vi "Stepper Mover.vi"() -> ()   [LabVIEW 2018]
doc: "Use this template to build a producer/consumer design pattern with events to produce queue items. Use this design pattern instead of the User Interface Event Handler pattern for user interfaces when you want to execute code asynchronously in response to an event without slowing the user interface responsiveness."
uses:
  publisher action.ctl
panel:
  in  "Instrument Address":refnum<visa-resource-name>="ASRL2::INSTR"
  in  "Tab Control":enum32{"main", "ignore"}(tab)
  in  "move-to pos!":dbl(slide)=743.9484386624194 scale=0.0..10000.0 scale format="%^#6_6g"
  out "current pos...":dbl(slide) scale=0.0..10000.0
  in  "set velocity!":i32=1001
  in  "Stop!":bool
  out "Moving..":bool
  in  "Init!":bool
  in  "Set to zero!":bool
  out "error out":errorcluster={"status"=TRUE, "code"=5202, "source"="Stepper Command Match"}
  out "Current Bottom Position":dbl format="%.4f"
  in  "Move to Bottom Position (deg or in)":dbl=10.41515984909622 format="%.4f"
  in  "Rotator":T1(ring)=enum."System B 50 mm Magnet"
  out "Timeout error":bool
  in  "Exit!":bool
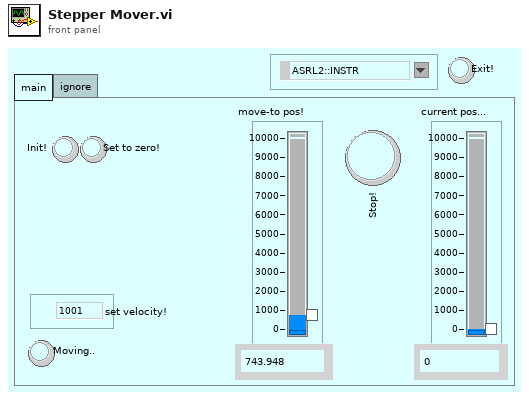
[diagram p1: front panel]
types:
  T1 = enum16{"Dilution Fridge SCM 1", "System A SCM 2", "System B 50 mm Magnet", "He-3 32 mm Magnet", "Portable Dil Fridge Rotator", "Linear Position", "System E Probe 1"}
  T2 = typedef "publisher action.ctl" = enum16{"set", "get"}
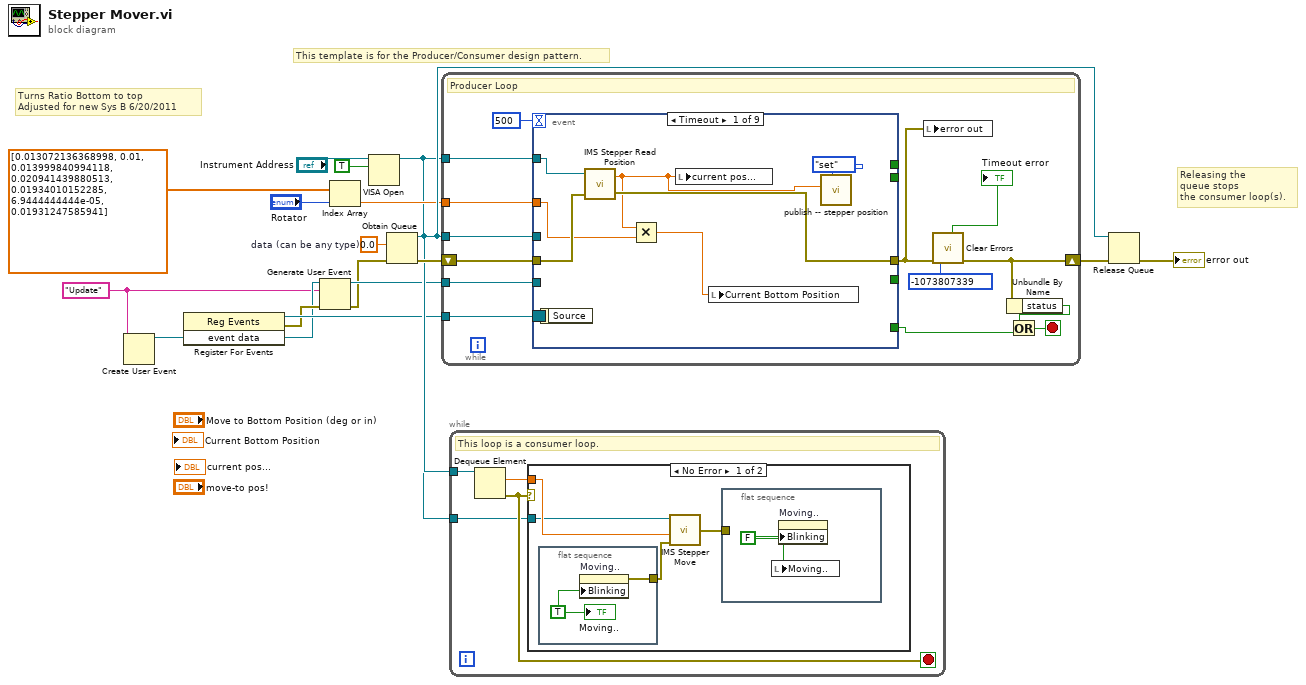
[diagram p0: block diagram]
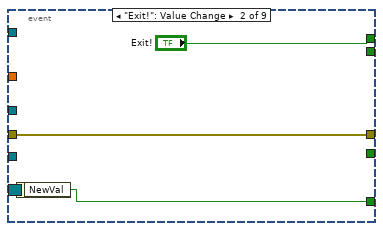
[diagram p3: hidden frame]
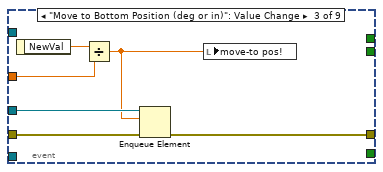
[diagram p4: hidden frame]
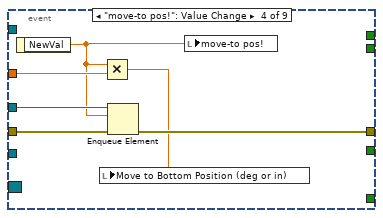
[diagram p5: hidden frame]
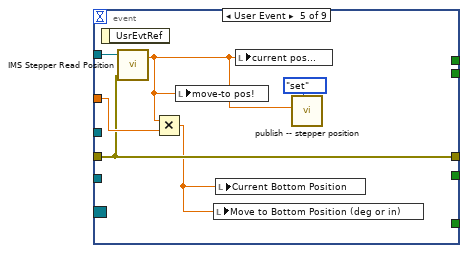
[diagram p6: hidden frame]
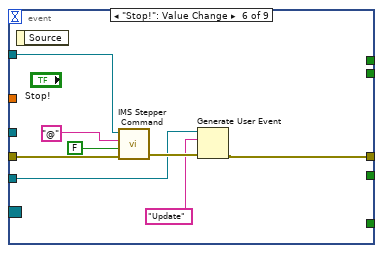
[diagram p7: hidden frame]
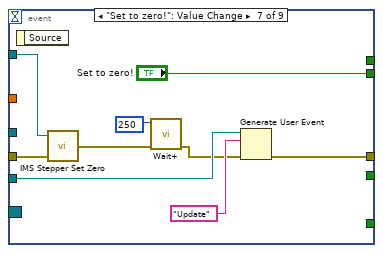
[diagram p8: hidden frame]
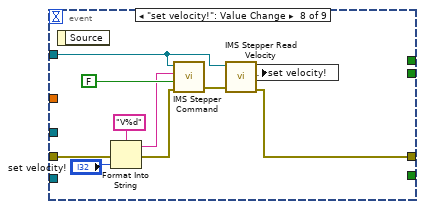
[diagram p9: hidden frame]
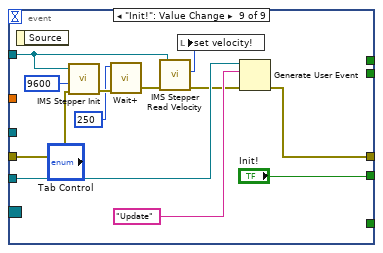
[diagram p10: hidden frame]
diagram:
  w2 = "Update" ("event data")
  w15 = 0.0  # data (can be any type)
  # "Turns Ratio Bottom to top\nAdjusted for new Sys B 6/20/2011"
  # "Releasing the\nqueue stops\nthe consumer loop(s)."
  # "This template is for the Producer/Consumer design pattern."
  n1 = Create User Event(user event datatype=w2) -> (user event=w5:refnum<user-event>)  [unwired: 1 in, 1 out]
  n2 = register-events(w5) -> (reference out=w7:refnum<event-registration>, error out=w6:errorcluster)  [unwired: 2 in]
  n3 = Generate User Event(user event=w5, event data cluster=w2, error in=w6) -> (user event out=w4:refnum<user-event>, error out=w3:errorcluster)  [unwired: 1 in]
  n4 = Index Array(array=dbl[] [0.013072136368998, 0.01, 0.013999840994118, 0.020941439880513, 0.01934010152285, 6.9444444444e-05, 0.01931247585941], index="Rotator") -> (element=w9:dbl)
  n5 = VISA Open(duplicate session (F)=TRUE, VISA resource name="Instrument Address") -> (VISA resource name=w8:refnum<visa-resource-name>)  [unwired: 3 in, 1 out]
  n6 = Obtain Queue(element data type=w15, error in (no error)=w3) -> (queue out=w14:refnum<queue>, error out=w17:errorcluster)  [unwired: 3 in, 1 out]
  n7 = while {
    shift-right: [w19] -> w16
    shift-left: w17 -> [w30]
    tunnel: w14 -> [w31]
    tunnel: w8 -> [w25]
    tunnel: w9 -> [w24]
    tunnel: w7 -> [w23]
    tunnel: w4 -> [w22]
    stop <- w28 stop-if-true
    # "Producer Loop"
    n8 = event shown="[0] Timeout" {
      selector: w23 -> [_ _ _ _ _ _ _ _ _]
      dyn-events: _ -> [_ _ _ _ _ _ _ _ _]
      timeout: 500 -> [_ _ _ _ _ _ _ _ _]
      tunnel: w31 -> [_ _ w47 w53 _ _ _ _ _]
      tunnel: w30 -> [w38 w41 w46 w52 w57 w65 w76 w82 w95]
      tunnel: [w35 w41 w45 w51 w57 w63 w74 w77 w98] -> w18
      tunnel: [_ w40 _ _ _ _ _ _ _] -> w29
      tunnel: w25 -> [w37 _ _ _ w58 w67 w75 w79 w92]
      tunnel: w24 -> [w36 _ w44 w50 w59 _ _ _ _]
      tunnel: w22 -> [_ _ _ _ _ w61 w73 _ w97]
      tunnel: [_ _ _ _ _ _ "Set to zero!" _ _] -> _
      tunnel: [_ _ _ _ _ _ _ _ "Init!"] -> _
      tunnel: [_ "Exit!" _ _ _ _ _ _ _] -> _
      event Timeout {
        n9 = event-data() -> ()  [unwired: 1 in, 1 out]
        n10 = call "IMS Stepper Read Position.vi"("error in (no error)"=w38, "Instrument Address"=w37) -> ("error out"=w35:errorcluster, "Response"=w33:dbl)  [unwired: 1 in]
        n11 = Multiply(x=w33, y=w36) -> (x*y=w34:dbl)
        n12 = local write "current pos..."(w33) -> ()
        n13 = local write "Current Bottom Position"(w34) -> ()
        n14 = call "publish -- stepper position.vi"("publisher action"=publisher_action."set", "stepper pos IN"=w33) -> ()  [unwired: 9 in, 1 out]
      }
      event "Exit!": Value Change {
        n15 = event-data() -> ("NewVal"=w40:bool)  [unwired: 1 in]
      }
      event "Move to Bottom Position (deg or in)": Value Change {
        n16 = event-data() -> ("NewVal"=w43:dbl)  [unwired: 1 in]
        n17 = Divide(x=w43, y=w44) -> (x/y=w42:dbl)
        n18 = Enqueue Element(queue=w47, element=w42, error in (no error)=w46) -> (error out=w45:errorcluster)  [unwired: 1 in, 2 out]
        n19 = local write "move-to pos!"(w42) -> ()
      }
      event "move-to pos!": Value Change {
        n20 = event-data() -> ("NewVal"=w48:dbl)  [unwired: 1 in]
        n21 = Multiply(x=w48, y=w50) -> (x*y=w49:dbl)
        n22 = local write "Move to Bottom Position (deg or in)"(w49) -> ()
        n23 = Enqueue Element(queue=w53, element=w48, error in (no error)=w52) -> (error out=w51:errorcluster)  [unwired: 1 in, 2 out]
        n24 = local write "move-to pos!"(w48) -> ()
      }
      event User Event {
        n25 = event-data() -> ()  [unwired: 1 in, 1 out]
        n26 = call "IMS Stepper Read Position.vi"("error in (no error)"=w57, "Instrument Address"=w58) -> ("Response"=w55:dbl)  [unwired: 1 in, 1 out]
        n27 = Multiply(x=w55, y=w59) -> (x*y=w56:dbl)
        n28 = local write "move-to pos!"(w55) -> ()
        n29 = local write "Move to Bottom Position (deg or in)"(w56) -> ()
        n30 = local write "Current Bottom Position"(w56) -> ()
        n31 = local write "current pos..."(w55) -> ()
        n32 = call "publish -- stepper position.vi"("publisher action"=publisher_action."set", "stepper pos IN"=w55) -> ()  [unwired: 9 in, 1 out]
      }
      event "Stop!": Value Change {
        n33 = event-data() -> ()  [unwired: 1 in, 1 out]
        n34 = call "IMS Stepper Command.vi"("Instrument Address"=w67, "Command"="@", "Mode"=FALSE, "error in (no error)"=w65) -> ("error out"=w62:errorcluster)  [unwired: 2 in, 2 out]
        n35 = Generate User Event(user event=w61, event data cluster="Update" ("event data"), error in=w62) -> (error out=w63:errorcluster)  [unwired: 1 in, 1 out]
      }
      event "Set to zero!": Value Change {
        n36 = event-data() -> ()  [unwired: 1 in, 1 out]
        n37 = call "IMS Stepper Set Zero.vi"("error in (no error)"=w76, "Instrument Address"=w75) -> ("error out"=w70:errorcluster)  [unwired: 1 in]
        n38 = call "Wait+.vi"("Error In"=w70, "milliseconds to wait"=u32 250) -> ("Error Out"=w69:errorcluster)  [unwired: 4 in, 1 out]
        n39 = Generate User Event(user event=w73, event data cluster="Update" ("event data"), error in=w69) -> (error out=w74:errorcluster)  [unwired: 1 in, 1 out]
      }
      event "set velocity!": Value Change {
        n40 = event-data() -> ()  [unwired: 1 in, 1 out]
        n41 = Format Into String(format string="V%d", error in=w82, "set velocity!") -> (resulting string=w83:string, error out=w81:errorcluster)  [unwired: 1 in]
        n42 = call "IMS Stepper Command.vi"("Instrument Address"=w79, "Command"=w83, "Mode"=FALSE, "error in (no error)"=w81) -> ("error out"=w80:errorcluster)  [unwired: 2 in, 2 out]
        n43 = call "IMS Stepper Read Velocity.vi"("error in (no error)"=w80, "Instrument Address"=w79) -> ("error out"=w77:errorcluster, "Velocity"=w78:i32)  [unwired: 3 in, 1 out]
        n44 = local write "set velocity!"(w78) -> ()
      }
      event "Init!": Value Change {
        n45 = event-data() -> ()  [unwired: 1 in, 1 out]
        n46 = call "IMS Stepper Init.vi"("error in (no error)"=w95, "Baud Rate"=u32 9600, "Instrument Address"=w92) -> ("error out"=w89:errorcluster)  [unwired: 1 in, 1 out]
        n47 = call "Wait+.vi"("Error In"=w89, "milliseconds to wait"=u32 250) -> ("Error Out"=w90:errorcluster)  [unwired: 4 in, 1 out]
        n48 = call "IMS Stepper Read Velocity.vi"("error in (no error)"=w90, "Instrument Address"=w92) -> ("error out"=w93:errorcluster, "Velocity"=w91:i32)  [unwired: 3 in, 1 out]
        n49 = local write "set velocity!"(w91) -> ()
        n50 = Generate User Event(user event=w97, event data cluster="Update" ("event data"), error in=w93) -> (error out=w98:errorcluster)  [unwired: 1 in, 1 out]
      }
    }
    n51 = local write "error out"(w18) -> ()
    n52 = call <vilib>:"Clear Errors.vi"("error in (no error)"=w18, "specific error code to clear (0: all)"=-1073807339) -> ("error out"=w19:errorcluster, "specific error cleared?"=→"Timeout error":bool)  [unwired: 4 in]
    n53 = Unbundle By Name(w19) -> ("status"=w27:bool)
    n54 = Or(x=w27, y=w29) -> (x .or. y?=w28:bool)
  }
  n55 = while {
    tunnel: w14 -> [w102]
    tunnel: w8 -> [w99]
    stop <- w101 stop-if-true
    # "This loop is a consumer loop."
    n56 = Dequeue Element(queue=w102) -> (element=w100:dbl, error out=w101:errorcluster)  [unwired: 2 in, 2 out]
    n57 = case shown="No Error" w101 {
      tunnel: w100 -> [w106 _]
      tunnel: w99 -> [w105 _]
      frame No Error {
        n58 = flat-sequence {
          tunnel: [w107] -> w104
          frame #0 {
            w108 = TRUE ("Moving")
            n59 = property on="Moving.." class="Bool (strict)"("Blinking"=w108) -> (error out=w107:errorcluster)  [unwired: 2 in, 1 out]
            "Moving.." <- w108
          }
        }
        n60 = call "IMS Stepper Move.vi"("Instrument Address"=w105, "Distance"=w106, "error in (no error)"=w104) -> ("error out"=w103:errorcluster)  [unwired: 2 in]
        n61 = flat-sequence {
          tunnel: w103 -> [_]
          frame #0 {
            w109 = FALSE ("Moving")
            n62 = local write "Moving.."(w109) -> ()
            n63 = property on="Moving.." class="Bool (strict)"("Blinking"=w109) -> ()  [unwired: 2 in, 2 out]
          }
        }
      }
      frame Error {
      }
    }
  }
  n64 = Release Queue(queue=w14, error in (no error)=w16) -> (error out=→"error out":errorcluster)  [unwired: 1 in, 2 out]
